vi "ROC_file_split.vi"(10 "数据存放路径":path) -> (2 "tdms out":refnum<k34>)   [LabVIEW 2017]
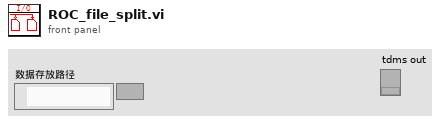
[diagram p1: front panel]
types:
  T1 = enum16{"open", "open or create", "create or replace", "create", "open (read-only)"}
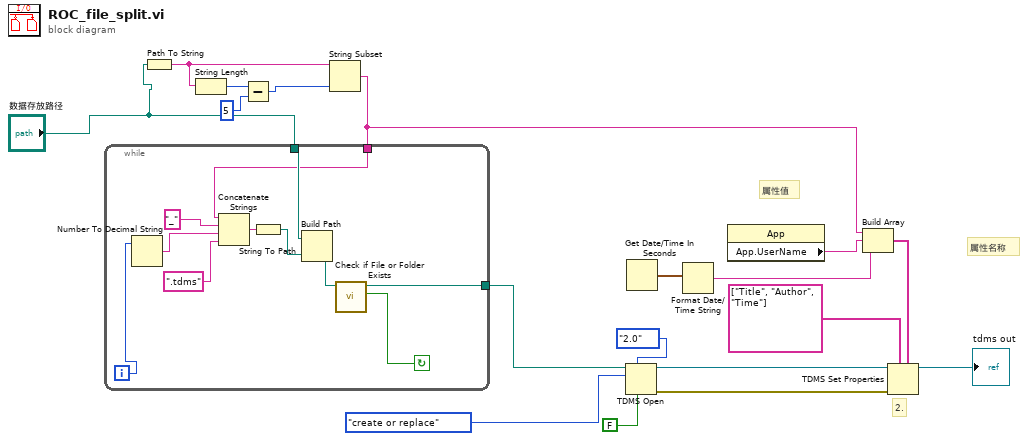
[diagram p0: block diagram]
diagram:
  # "属性名称"
  # "属性值"
  # "2."
  n1 = Path To String(path="数据存放路径") -> (string=w6:string)
  n2 = String Length(string=w6) -> (length=w5:i32)
  n3 = Subtract(x=w5, y=5) -> (x-y=w3:i32)
  n4 = String Subset(string=w6, length (rest)=w3) -> (substring=w1:string)  [unwired: 1 in]
  n5 = while {
    tunnel: "数据存放路径" -> [w26]
    tunnel: [w21] -> w2
    tunnel: w1 -> [w19]
    i -> [w23]
    stop <- w25 continue-if-true
    n6 = Number To Decimal String(number=w23) -> (decimal integer string=w22:string)  [unwired: 1 in]
    n7 = Concatenate Strings(w19, "_" ("string"), w22, ".tdms" ("字符串")) -> (w28:string)
    n8 = String To Path(string=w28) -> (path=w29:path)
    n9 = Build Path(base path=w26, name or relative path=w29) -> (appended path=w27:path)
    n10 = call <vilib>:"Check if File or Folder Exists.vi"("path"=w27) -> ("file or folder exists?"=w25:bool, "dup path"=w21:path)  [unwired: 8 in, 1 out]
  }
  n11 = TDMS Open(6:FALSE ("disable buffering (T)"), 7:enum16{"1.0", "2.0"}."2.0" ("file format version (2.0)"), 10:T1."create or replace" ("operation"), 11:w2) -> (0:w15:errorcluster, 3:w14:refnum<k34>)  [unwired: 3 in]
  n12 = Get Date/Time In Seconds() -> (seconds since 1Jan1904=w17:timestamp)
  n13 = Format Date/Time String(seconds (now)=w17) -> (date/time string=w18:string)  [unwired: 2 in]
  n14 = property class="App"() -> ("App.UserName"=w12:string)  [unwired: 2 in, 2 out]
  n15 = Build Array(w1, w12, w18) -> (w13:string[])
  n16 = TDMS Set Properties(5:w13, 7:string[] ["Title", "Author", "Time"] ("property names"), 8:w15, 11:w14) -> (3:→"tdms out":refnum<k34>)  [unwired: 5 out]
